vi "rs3 get stream profile data.vi"(8 "error in (no error)":errorcluster, 11 "Profile":u64) -> (0 "error out":errorcluster, 1 "index":i32, 2 "error out":u64, 3 "Profile out":u64, 4 "frame rate":i32, 5 "unique id":i32, 6 "RS Format":u16(ring)=6 items=["    RS2_FORMAT_ANY             , /**< When passed to enable stream, librealsense will try to provide best suited format */", "    RS2_FORMAT_Z16             , /**< 16-bit linear depth values. The depth is meters is equal to depth scale * pixel value. */", "    RS2_FORMAT_DISPARITY16     , /**< 16-bit linear disparity values. The depth in meters is equal to depth scale / pixel value. */", "    RS2_FORMAT_XYZ32F          , /**< 32-bit floating point 3D coordinates. */", "    RS2_FORMAT_YUYV            , /**< Standard YUV pixel format as described in https://en.wikipedia.org/wiki/YUV */", "    RS2_FORMAT_RGB8            , /**< 8-bit red, green and blue channels */", "    RS2_FORMAT_BGR8            , /**< 8-bit blue, green, and red channels -- suitable for OpenCV */", "    RS2_FORMAT_RGBA8           , /**< 8-bit red, green and blue channels + constant alpha channel equal to FF */", "    RS2_FORMAT_BGRA8           , /**< 8-bit blue, green, and red channels + constant alpha channel equal to FF */", "    RS2_FORMAT_Y8              , /**< 8-bit per-pixel grayscale image */", "    RS2_FORMAT_Y16             , /**< 16-bit per-pixel grayscale image */", "    RS2_FORMAT_RAW10           , /**< Four 10-bit luminance values encoded into a 5-byte macropixel */", "    RS2_FORMAT_RAW16           , /**< 16-bit raw image */", "    RS2_FORMAT_RAW8            , /**< 8-bit raw image */", "    RS2_FORMAT_UYVY            , /**< Similar to the standard YUYV pixel format, but packed in a different order */", "    RS2_FORMAT_MOTION_RAW      , /**< Raw data from the motion sensor */", "    RS2_FORMAT_MOTION_XYZ32F   , /**< Motion data packed as 3 32-bit float values, for X, Y, and Z axis */", "    RS2_FORMAT_GPIO_RAW        , /**< Raw data from the external sensors hooked to one of the GPIO's */", "    RS2_FORMAT_COUNT             /**< Number of enumeration values. Not a valid input: intended to be used in for-loops. */"], 7 "RS Stream":u16(ring) items=["    RS2_STREAM_ANY,", "    RS2_STREAM_DEPTH                            , /**< Native stream of depth data produced by RealSense device */", "    RS2_STREAM_COLOR                            , /**< Native stream of color data captured by RealSense device */", "    RS2_STREAM_INFRARED                         , /**< Native stream of infrared data captured by RealSense device */", "    RS2_STREAM_FISHEYE                          , /**< Native stream of fish-eye (wide) data captured from the dedicate motion camera */", "    RS2_STREAM_GYRO                             , /**< Native stream of gyroscope motion data produced by RealSense device */", "    RS2_STREAM_ACCEL                            , /**< Native stream of accelerometer motion data produced by RealSense device */", "    RS2_STREAM_GPIO                             , /**< Signals from external device connected through GPIO */", "    RS2_STREAM_COUNT"])   [LabVIEW 2019, in "libRealSense3.lvlib"]
doc: "Returns the information about a specific selected PROFILE. \n\nINPUT:\nProfile This is the handle to the profile data\n\nOUTPUT: \ninfo stream, format, index, unique ID, frame rate, and error\n\nNote that certain combinations exist to uniquely define a stream. For example\nstream=depth, format=Z16, index=0 This is the depth stream\nstream=IR, format=RGB8, index=0 This is the left color camera of a D410/D415 camera\nstream=IR, format=Y8, index=1 This is the LEFT monochrome camera stream\nstream=IR, format=Y8, index=2 This the the RIGHT monochome camera stream"
uses:
  libRealSense3.lvlib
  realsense2.dll
panel:
  # "RS3 Get Stream Profile Data"
  # "(C) Intel Corp 2017.,  AGJ"
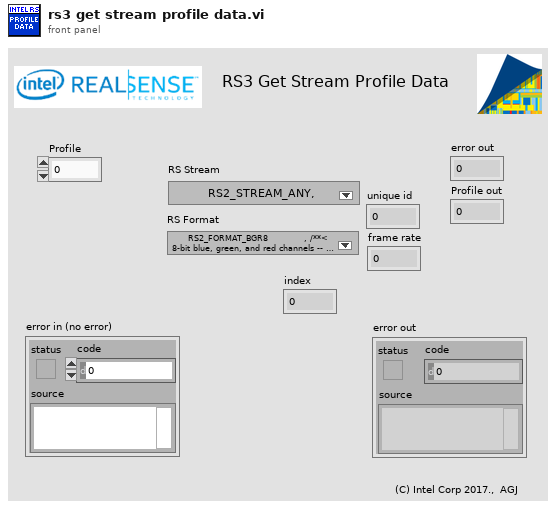
[diagram p1: front panel]
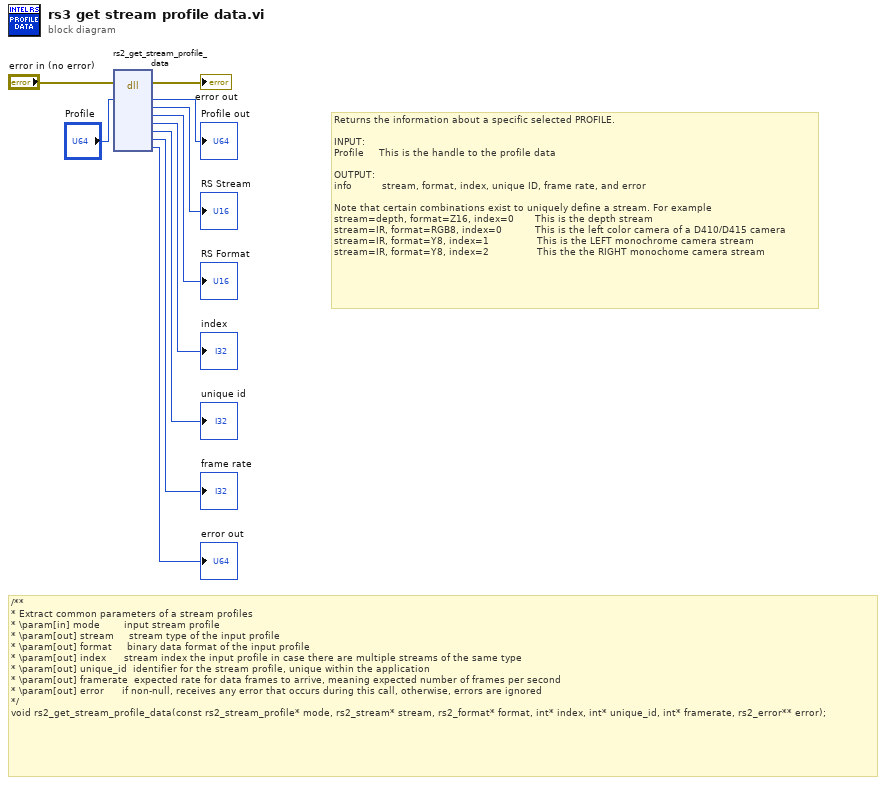
[diagram p0: block diagram]
diagram:
  # "Returns the information about a specific selected PROFILE. \n\nINPUT:\nProfile     This is the handle to the profile data\n\nOUTPUT: \ninfo          stream, format, index, unique ID, frame rate, and error\n\nNote that certain combinations exist to uniquely define a stream. For example\nstream=depth, format=Z16, index=0       This is the depth stream\nstream=IR, format=RGB8, index=0           This is the left color camera of a D410/D415 camera\nstream=IR, format=Y8, index=1                This is the LEFT monochrome camera stream\nstream=IR, format=Y8, index=2                This the the RIGHT monochome camera stream"
  # "/**\n* Extract common parameters of a stream profiles\n* \\param[in] mode        input stream profile\n* \\param[out] stream     stream type of the input profile\n* \\param[out] format     binary data format of the input profile\n* \\param[out] index      stream index the input profile in case there are multiple streams of the same type\n* \\param[out] unique_id  identifier for the stream profile, unique within the application\n* \\param[out] framerate  expected rate for data frames to arrive, meaning expected number of frames per second\n* \\param[out] error      if non-null, receives any error that occurs during this call, otherwise, errors are ignored\n*/\nvoid rs2_get_stream_profile_data(const rs2_stream_profile* mode, rs2_stream* stream, rs2_format* format, int* index, int* unique_id, int* framerate, rs2_error** error);"
  n1 = dll-call lib="C:/SmartekVision/Projects/RS-D4-ETH/Software/RS-SDK/wrappers/labview/realsense2.dll" fn="rs2_get_stream_profile_data"(error in="error in (no error)", "Profile"="Profile") -> (error out=→"error out":errorcluster, "Profile"=→"Profile out":u64, "stream"=→"RS Stream":u32, "format"=→"RS Format":u32, "index"=→"index":i32, "unique id"=→"unique id":i32, "frame rate"=→"frame rate":i32, "error"=→"error out":u64)  [unwired: 9 in, 1 out]
